vi "CheckAllTouchSensors.vi"(5 "Touch sensor lines":T1={"Home touch"=3, "Touch 1"=1, "Touch 2"=2, "Touch 3"=4, "Touch 4"=4}, 6 "DI Task":refnum<k21>) -> (0 "TS 4":bool, 1 "TS 3":bool, 2 "TS 2":bool, 3 "TS 1":bool, 4 "Home?":bool)   [LabVIEW 2010]
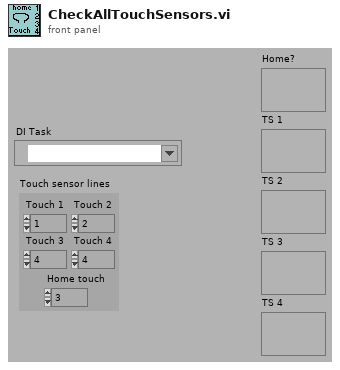
[diagram p1: front panel]
types:
  T1 = cluster{"Home touch":i16, "Touch 1":i16, "Touch 2":i16, "Touch 3":i16, "Touch 4":i16}
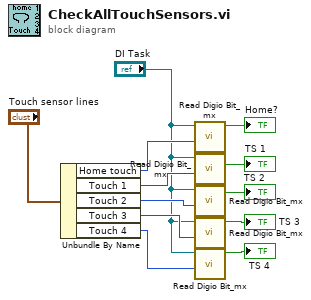
[diagram p0: block diagram]
diagram:
  n1 = Unbundle By Name("Touch sensor lines") -> ("Home touch"=w11:i16, "Touch 1"=w9:i16, "Touch 2"=w7:i16, "Touch 3"=w6:i16, "Touch 4"=w4:i16)
  n2 = call "Read Digio Bit_mx.vi"("line"=w11, "DI Task"="DI Task") -> ("line state"=→"Home?":bool)  [unwired: 7 in, 1 out]
  n3 = call "Read Digio Bit_mx.vi"("line"=w9, "DI Task"="DI Task") -> ("line state"=→"TS 1":bool)  [unwired: 7 in, 1 out]
  n4 = call "Read Digio Bit_mx.vi"("line"=w7, "DI Task"="DI Task") -> ("line state"=→"TS 2":bool)  [unwired: 7 in, 1 out]
  n5 = call "Read Digio Bit_mx.vi"("line"=w6, "DI Task"="DI Task") -> ("line state"=→"TS 3":bool)  [unwired: 7 in, 1 out]
  n6 = call "Read Digio Bit_mx.vi"("line"=w4, "DI Task"="DI Task") -> ("line state"=→"TS 4":bool)  [unwired: 7 in, 1 out]
